vi "Write Channel Interface.vi"(8 "error in (no error)":errorcluster, 10 "Channel Interface":T1={"Coupling"=0, "Differential Input"=FALSE, "Direct-to-ADC"=FALSE, "Range"=2000, "Impedance"=50, "DC Offset"=0, "Filter"=0} {"Impedance" min=50 max=1000000 step=999950; "Coupling" items=["DC", "AC"]}, 11 "Control_interface in":refnum<class "Control_interface.lvclass">) -> (0 "error out":errorcluster, 3 "Control_interface out":refnum<class "Control_interface.lvclass">)   [LabVIEW 2015, in "Control_interface.lvclass"]
uses:
  Control_interface.lvclass
  Control_interface.lvclass/Control_interface.ctl
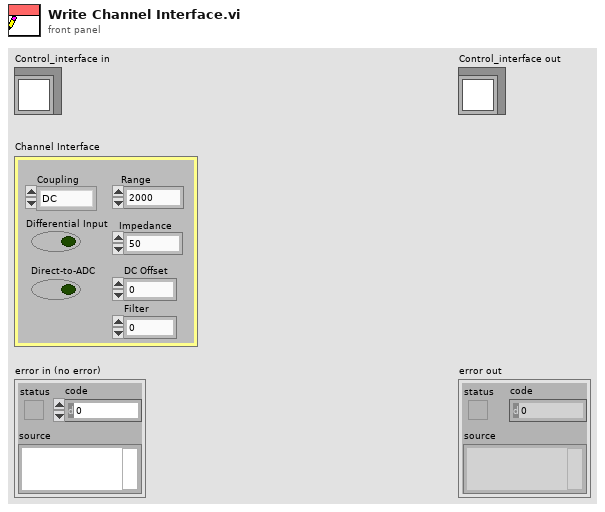
[diagram p1: front panel]
types:
  T1 = cluster{"Coupling":u16, "Differential Input":bool, "Direct-to-ADC":bool, "Range":u32, "Impedance":u32, "DC Offset":i32, "Filter":i32}
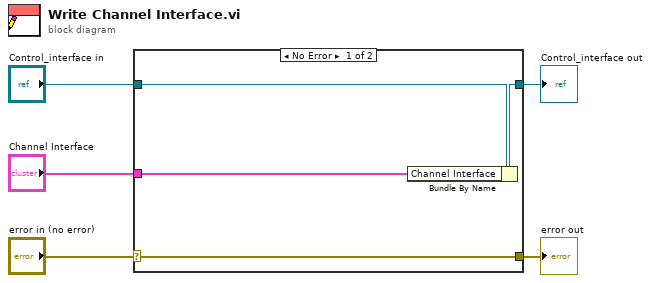
[diagram p0: block diagram]
diagram:
  n1 = case shown="No Error" "error in (no error)" {
    selector: "error in (no error)" -> [w9 w10]
    tunnel: [w9 w10] -> w4
    tunnel: [w7 w11] -> w2
    tunnel: "Control_interface in" -> [w8 w11]
    tunnel: "Channel Interface" -> [w6 _]
    frame No Error {
      n2 = Bundle By Name(cluster=w8, "Channel Interface"=w6) -> (w7:refnum<class "Control_interface.lvclass">)
    }
    frame Error {
    }
  }
  "error out" <- w4
  "Control_interface out" <- w2
